vi "custom_trajectories.vi"() -> ()   [LabVIEW 2015]
panel:
  in  "custom_trajectory":dbl[](array[numeric])
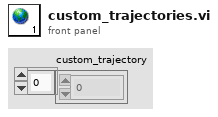
[diagram p1: front panel]
diagram:
